vi "Get ID.vi"(8 "error in (no error)":errorcluster, 11 "FW102C in":i32) -> (0 "error out":errorcluster, 2 "ID":string, 3 "FW102C out":i32)   [LabVIEW 2020, in "Thorlabs_FW102C.lvlib"]
uses:
  Thorlabs_FW102C.lvlib
  Library/FilterWheel102_win32.dll
  Library/FilterWheel102_win64.dll
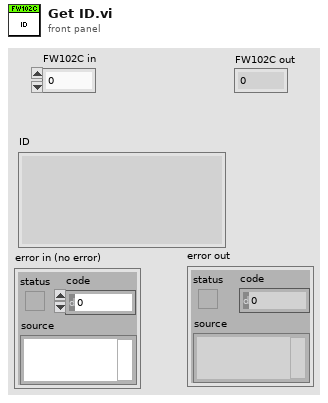
[diagram p1: front panel]
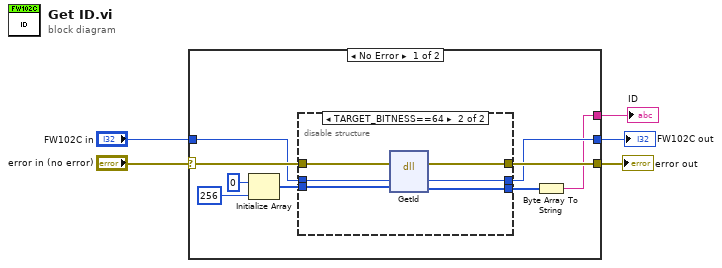
[diagram p0: block diagram]
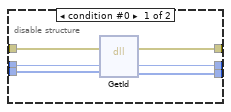
[diagram p2: hidden frame]
diagram:
  n1 = case shown="No Error" "error in (no error)" {
    selector: "error in (no error)" -> [w14 w27]
    tunnel: [w13 w27] -> w5
    tunnel: "FW102C in" -> [w12 w28]
    tunnel: [w6 _] -> w2
    tunnel: [w11 w28] -> w1
    frame No Error {
      n2 = Initialize Array(u8 0 ("element"), 256 ("dimension size")) -> (w7:u8[])
      n3 = disable-structure shown="TARGET_BITNESS==64" {
        disable-tunnel: w14 -> [w20 w26]
        disable-tunnel: [w19 w25] -> w13
        disable-tunnel: w12 -> [w18 w24]
        disable-tunnel: [w17 w23] -> w11
        disable-tunnel: [w16 w22] -> w10
        disable-tunnel: w7 -> [w15 w21]
        frame condition #0 {
          n4 = dll-call lib="C:/Users/astrolab/Desktop/Peter_Ferguson/TCal/Labview_Code/Other_Libraries/Thorlabs_FW102C/Library/FilterWheel102_win32.dll" fn="GetId"(error in=w20, "hdl"=w18, "id"=w15) -> (error out=w19:errorcluster, "hdl"=w17:i32, "id"=w16:u8[])  [unwired: 3 in, 1 out]
        }
        frame condition #1 (active) {
          n5 = dll-call lib="C:/Users/astrolab/Desktop/Peter_Ferguson/TCal/Labview_Code/Other_Libraries/Thorlabs_FW102C/Library/FilterWheel102_win64.dll" fn="GetId"(error in=w26, "hdl"=w24, "id"=w21) -> (error out=w25:errorcluster, "hdl"=w23:i32, "id"=w22:u8[])  [unwired: 3 in, 1 out]
        }
      }
      n6 = Byte Array To String(unsigned byte array=w10) -> (string=w6:string)
    }
    frame Error {
    }
  }
  "error out" <- w5
  "ID" <- w2
  "FW102C out" <- w1
